vi "currentHostPC.vi"() -> ()   [LabVIEW 2020]
uses:
  <vilib>/Analysis/3filter.llb/Equi-Ripple BandPass (DBL).vi
  <vilib>/Analysis/NI_AALBase.lvlib
  <vilib>/gmath/NI_Gmath.lvlib
panel:
  out "Current 2":dbl[](graph)
  in  "Low/High current mode":bool
  out "Zero":dbl format="%#_6p"
  in  "Acquire Zero":bool
  in  "TIA 2":dbl
  out "Current":dbl format="%#_6p"
  in  "1/R2":dbl
  in  "1/R1":dbl
  out "Average TIA 3":dbl
  out "Average TIA 2":dbl
  out "Average TIA 1":dbl
  in  "percent (trim)":dbl=25.0
  in  "milliseconds to wait":u32=10
  out "Histogram Graph":T1(graph)
  out "Current":dbl(graph)
  in  "stop":bool
  out "TIA":T2(graph)
  out "Currrent State TIA 3":dbl
  out "Currrent State TIA 2":dbl
  out "Currrent State TIA 1":dbl
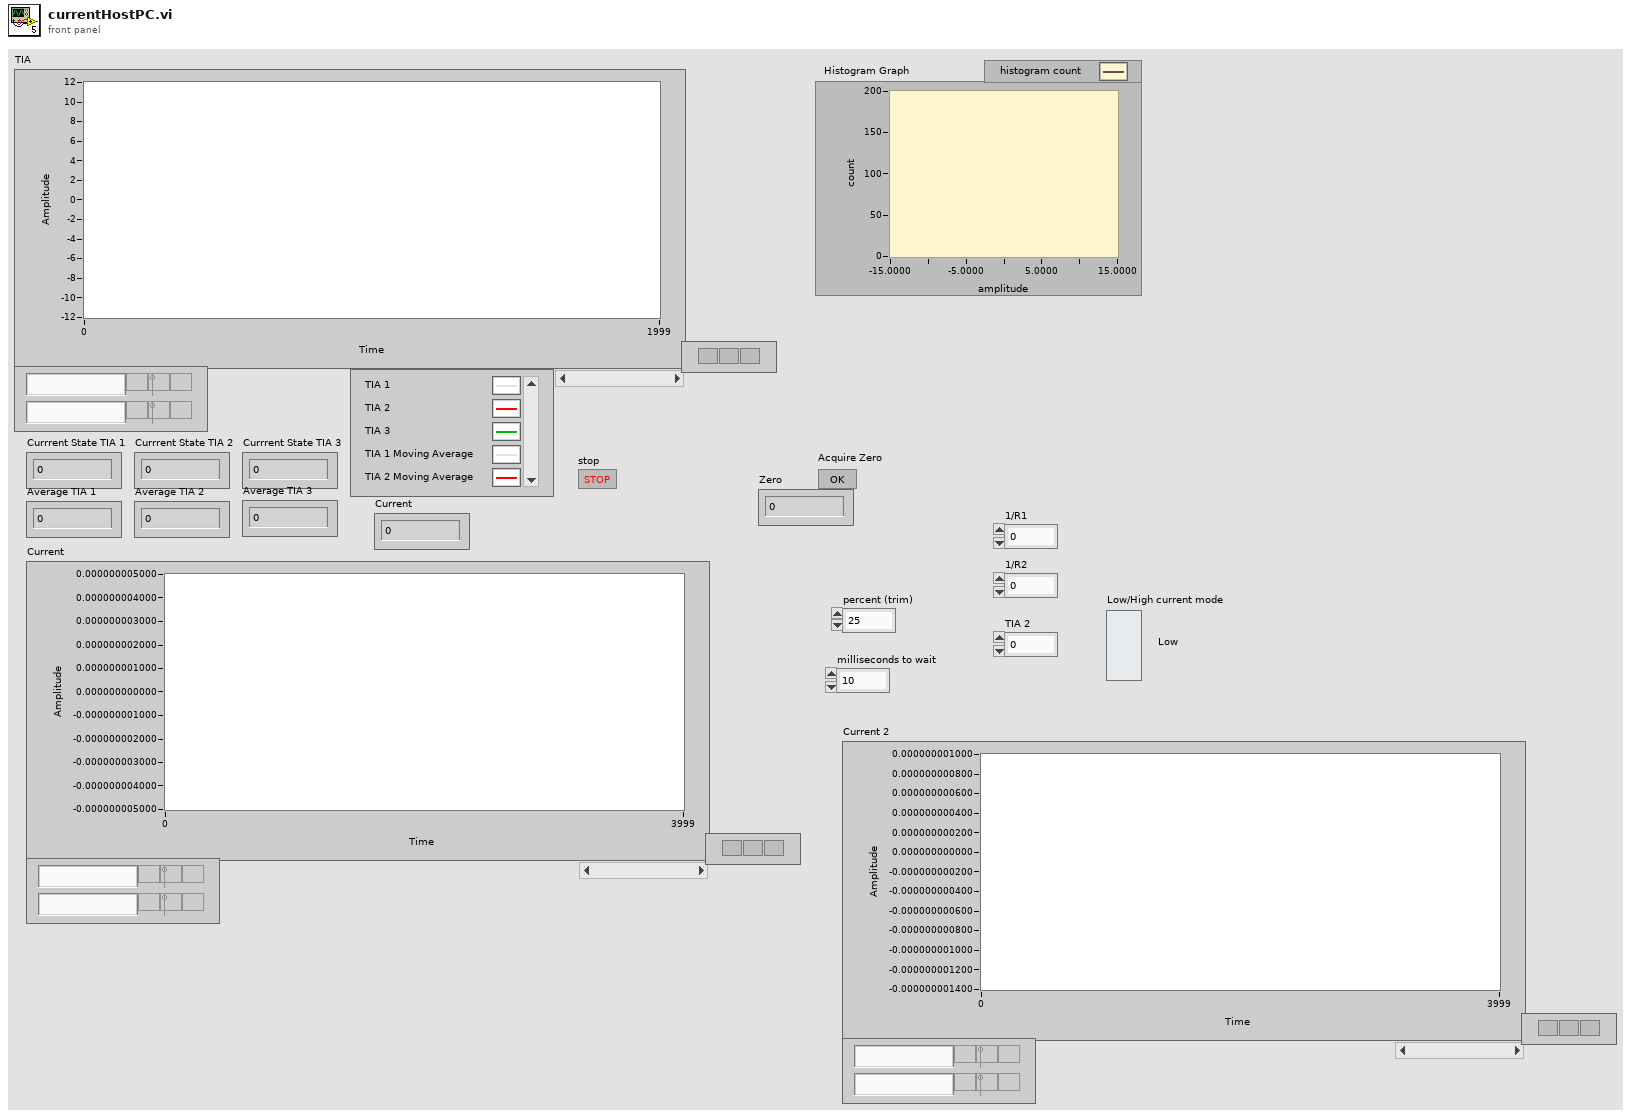
[diagram p1: front panel]
types:
  T1 = cluster{"X Values":dbl[], "Histogram: h(x)":i32[]}
  T2 = cluster{"Double":dbl, dbl, "Double":dbl, "mean value":dbl, "mean value":dbl, "mean value":dbl}
  T3 = enum16{"open", "replace", "create", "open or create", "replace or create", "replace or create with confirmation"}
  T4 = cluster{"Double":dbl, "Double":dbl, "Double":dbl, "mean value":dbl, "mean value":dbl, "mean value":dbl}
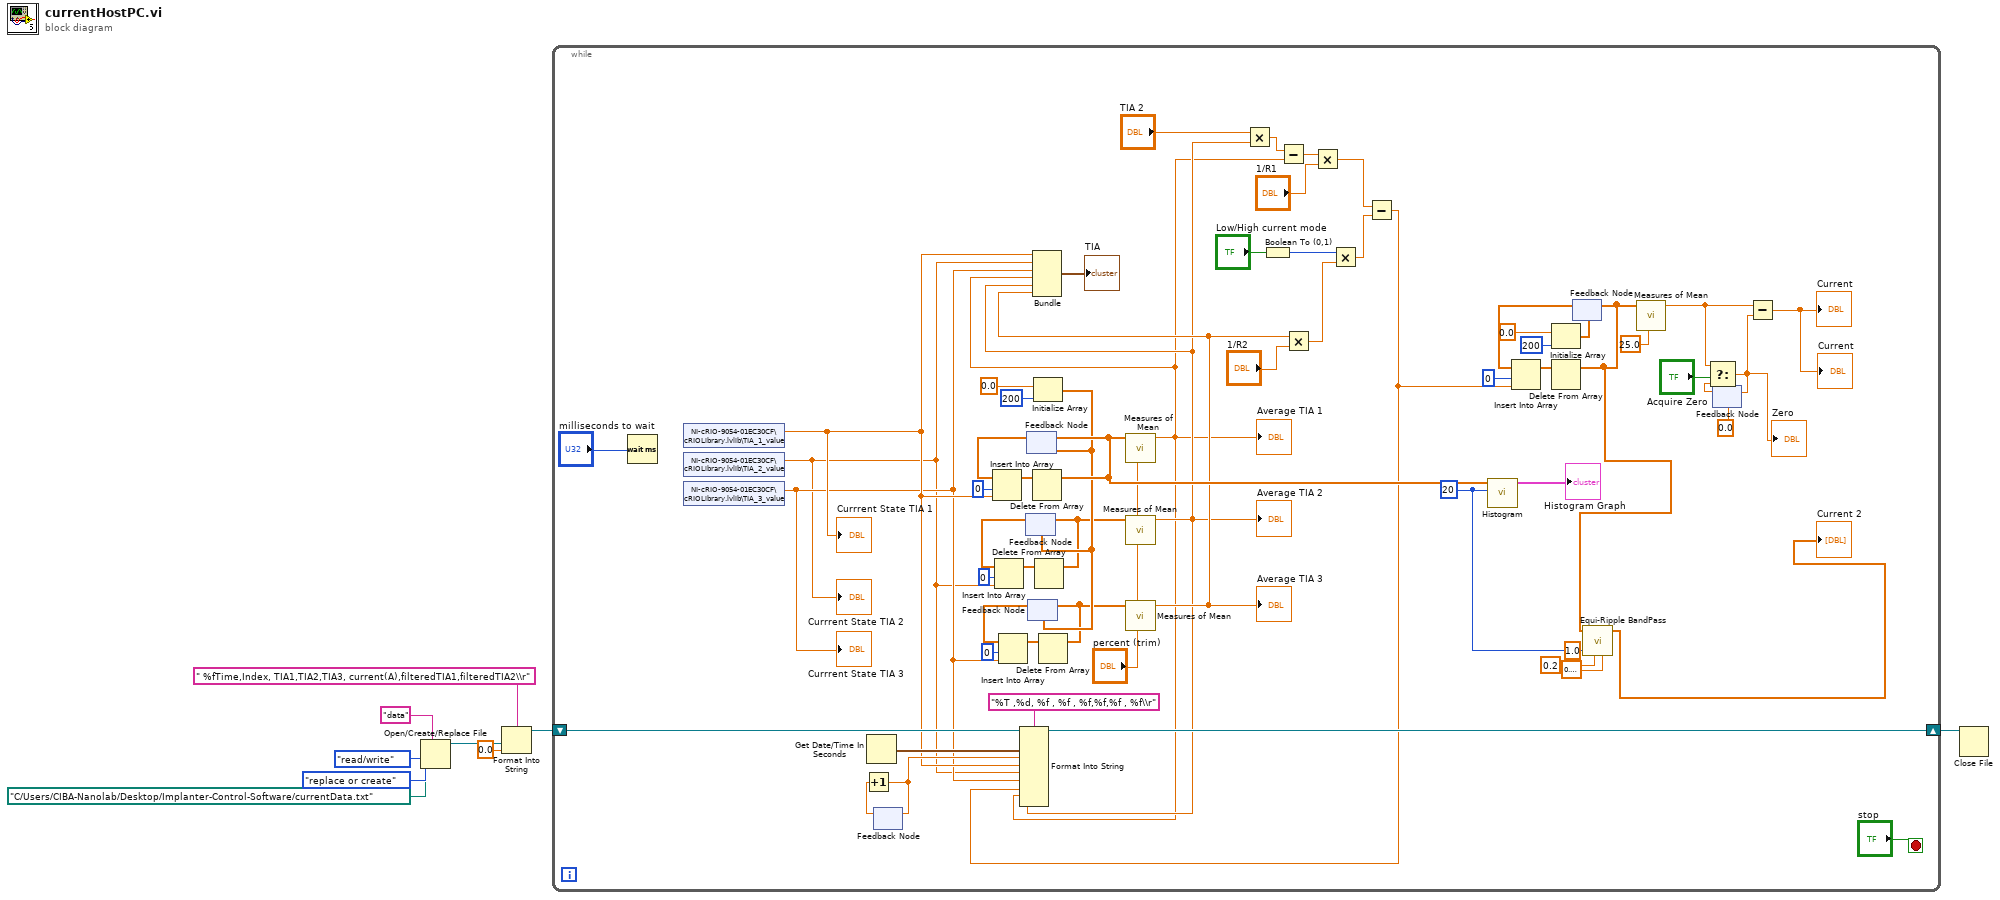
[diagram p0: block diagram]
diagram:
  n1 = Open/Create/Replace File(file path (use dialog)=path "C:/Users/CIBA-Nanolab/Desktop/Implanter-Control-Software/currentData.txt", prompt="data", operation (0:open)=T3."replace or create", access (0:read/write)=enum16{"read/write", "read-only", "write-only"}."read/write") -> (refnum out=w4:refnum<file>)  [unwired: 2 in, 2 out]
  n2 = Format Into String(format string=" %fTime,Index, TIA1,TIA2,TIA3, current(A),filteredTIA1,filteredTIA2\\r", initial string=w4, 0.0 ("input 1")) -> (resulting string=w3:refnum<file>)  [unwired: 1 in, 1 out]
  n3 = while {
    shift-right: [w68] -> w2
    shift-left: w3 -> [w69]
    stop <- "stop" stop-if-true
    w15 = 20
    n4 = Wait (ms)(milliseconds to wait="milliseconds to wait") -> ()  [unwired: 1 out]
    n5 = shared-variable "NI-cRIO-9054-01EC30CF\\cRIOLibrary.lvlib\\TIA_1_value"() -> (w61:dbl)  [unwired: 1 in, 1 out]
    "Currrent State TIA 1" <- w61
    n6 = shared-variable "NI-cRIO-9054-01EC30CF\\cRIOLibrary.lvlib\\TIA_2_value"() -> (w33:dbl)  [unwired: 1 in, 1 out]
    "Currrent State TIA 2" <- w33
    n7 = shared-variable "NI-cRIO-9054-01EC30CF\\cRIOLibrary.lvlib\\TIA_3_value"() -> (w43:dbl)  [unwired: 1 in, 1 out]
    "Currrent State TIA 3" <- w43
    n8 = Get Date/Time In Seconds() -> (seconds since 1Jan1904=w67:timestamp)
    n9 = feedback #1() -> (w65:dbl)  [unwired: 1 in]
    n10 = Increment(x=w65) -> (x+1=w64:dbl)
    n11 = feedback-in #1(w64) -> ()
    n12 = Initialize Array(0.0 ("element"), 200 ("dimension size")) -> (w42:dbl[])
    n13 = feedback #2(w42) -> (w55:dbl[])
    n14 = Insert Into Array(array=w55, index=0, new element=w33) -> (w57:dbl[])
    n15 = feedback #3(w42) -> (w62:dbl[])
    n16 = Insert Into Array(array=w62, index=0, new element=w61) -> (w63:dbl[])
    n17 = feedback #4(w42) -> (w44:dbl[])
    n18 = Insert Into Array(array=w44, index=0, new element=w43) -> (w46:dbl[])
    n19 = Delete From Array(array=w63) -> (array with subset deleted=w47:dbl[])  [unwired: 2 in, 1 out]
    n20 = feedback-in #3(w47) -> ()
    n21 = Delete From Array(array=w57) -> (array with subset deleted=w40:dbl[])  [unwired: 2 in, 1 out]
    n22 = feedback-in #2(w40) -> ()
    n23 = Delete From Array(array=w46) -> (array with subset deleted=w41:dbl[])  [unwired: 2 in, 1 out]
    n24 = feedback-in #4(w41) -> ()
    n25 = call <vilib>:"Measures of Mean.vi"("percent (trim)"="percent (trim)", "x array"=w47) -> ("mean value"=w21:dbl)  [unwired: 8 in, 1 out]
    "Average TIA 1" <- w21
    n26 = call <vilib>:"Measures of Mean.vi"("percent (trim)"="percent (trim)", "x array"=w40) -> ("mean value"=w30:dbl)  [unwired: 8 in, 1 out]
    "Average TIA 2" <- w30
    n27 = call <vilib>:"Measures of Mean.vi"("percent (trim)"="percent (trim)", "x array"=w41) -> ("mean value"=w32:dbl)  [unwired: 8 in, 1 out]
    "Average TIA 3" <- w32
    n28 = Bundle("Double"=w61, "Double"=w33, "Double"=w43, "mean value"=w21, "mean value"=w30, "mean value"=w32) -> (→"TIA":T4)  [unwired: 1 in]
    n29 = Multiply(x="TIA 2", y=w30) -> (x*y=w29:dbl)
    n30 = Boolean To (0,1)(Boolean="Low/High current mode") -> (0, 1=w18:i16)
    n31 = Subtract(x=w29, y=w21) -> (x-y=w38:dbl)
    n32 = Multiply(x=w32, y="1/R2") -> (x*y=w20:dbl)
    n33 = Multiply(x=w38, y="1/R1") -> (x*y=w37:dbl)
    n34 = Multiply(x=w18, y=w20) -> (x*y=w19:dbl)
    n35 = Subtract(x=w37, y=w19) -> (x-y=w36:dbl)
    n36 = Format Into String(format string="%T ,%d, %f , %f , %f,%f,%f , %f\\r", initial string=w69, w67, w64, w61, w33, w43, w36, w21, w30) -> (resulting string=w68:refnum<file>)  [unwired: 1 in, 1 out]
    n37 = call <vilib>:"Histogram.vi"("intervals"=w15, "X"=w47) -> ("Histogram Graph"=→"Histogram Graph":T1)  [unwired: 6 in, 3 out]
    n38 = Initialize Array(0.0 ("element"), 200 ("dimension size")) -> (w16:dbl[])
    n39 = feedback #5(w16) -> (w49:dbl[])
    n40 = Insert Into Array(array=w49, index=0, new element=w36) -> (w53:dbl[])
    n41 = Delete From Array(array=w53) -> (array with subset deleted=w11:dbl[])  [unwired: 2 in, 1 out]
    n42 = feedback-in #5(w11) -> ()
    n43 = call-poly <vilib>:"Equi-Ripple BandPass.vi"("X"=w11, "# of taps"=w15, "lower stop freq"=0.2, "higher stop freq"=0.4000000000000001, "sampling freq: fs"=1.0) -> ("Filtered X"=→"Current 2":dbl[])  [unwired: 3 in, 1 out]
    n44 = call <vilib>:"Measures of Mean.vi"("percent (trim)"=25.0, "x array"=w11) -> ("mean value"=w25:dbl)  [unwired: 8 in, 1 out]
    n45 = feedback #6(0.0 ("mean value")) -> (w26:dbl)
    n46 = Select(t=w25, s="Acquire Zero", f=w26) -> (s? t:f=w23:dbl)
    "Zero" <- w23
    n47 = feedback-in #6(w23) -> ()
    n48 = Subtract(x=w25, y=w23) -> (x-y=→"Current" →"Current":dbl)
  }
  n49 = Close File(refnum=w2) -> ()  [unwired: 1 in, 2 out]
